vi "Status Created Queues.vi"(11 "qqqqq in":refnum<class "qqqqq.lvclass">) -> (0 "Created Queue Count":i32, 1 "Created Queue Aliases":string[](array[string]), 2 "Created Queue Exist?":bool, 3 "qqqqq out":refnum<class "qqqqq.lvclass">)   [LabVIEW 2021, in "jettl Tools.lvlib" / "qqqqq.lvlib" / "qqqqq.lvclass"]
uses:
  qqqqq.lvclass
  qqqqq.lvclass/qqqqq.ctl
  jettl/Queue/Queue.lvclass
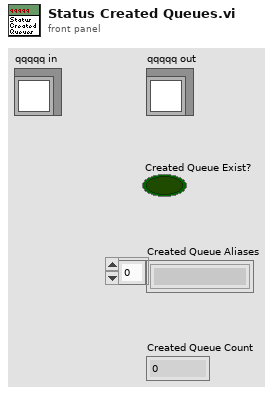
[diagram p1: front panel]
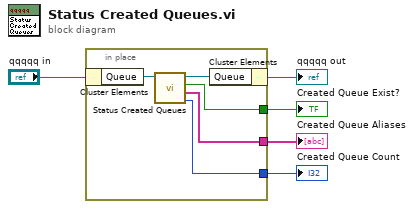
[diagram p0: block diagram]
diagram:
  n1 = in-place {
    in-place-border: [w8] -> w3
    in-place-border: [w7] -> w2
    in-place-border: [w6] -> w1
    n2 = in-place-cluster #1("qqqqq in") -> ("Queue"=w10:refnum<class "Queue.lvclass">)
    n3 = call-dynamic "Status Created Queues.vi"("Queue in"=w10) -> ("Created Queue Count"=w6:i32, "Created Queue Aliases"=w7:string[], "Created Queue Exist?"=w8:bool, "Queue out"=w9:refnum<class "Queue.lvclass">)  [unwired: 7 in]
    n4 = in-place-cluster #1("Queue"=w9) -> (→"qqqqq out":refnum<class "qqqqq.lvclass">)
  }
  "Created Queue Exist?" <- w3
  "Created Queue Aliases" <- w2
  "Created Queue Count" <- w1
